vi "ccdIsOpen.vi"() -> ()   [LabVIEW 2023, in "CCD.lvclass"]
uses:
  CCD.lvclass
  CCD.lvclass/CCD.ctl
  d9b87029-586e-44ee-a6e5-d4a5e0edce38.vi
  Communicator/Communicator.lvclass
  b59fd1e7-dcda-425c-bd6c-61aafb79e7f4.vi
  GenericDevice/GenericDevice.lvclass
  ccdIsOpen.ctl
panel:
  out "CCD is open?":T1
  out "CCD out":refnum<class "CCD.lvclass">
  in  "CCD in":refnum<class "CCD.lvclass">
  out "error out":errorcluster
  in  "error in (no error)":errorcluster
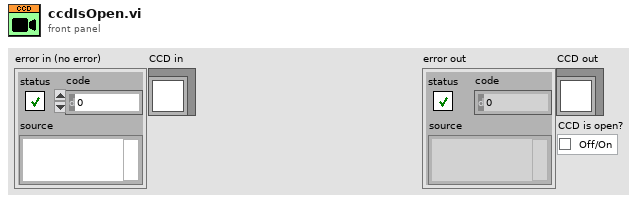
[diagram p1: front panel]
types:
  T1 = typedef "CCD.lvclass/ccdIsOpen.ctl" = cluster{"Checkbox":bool}
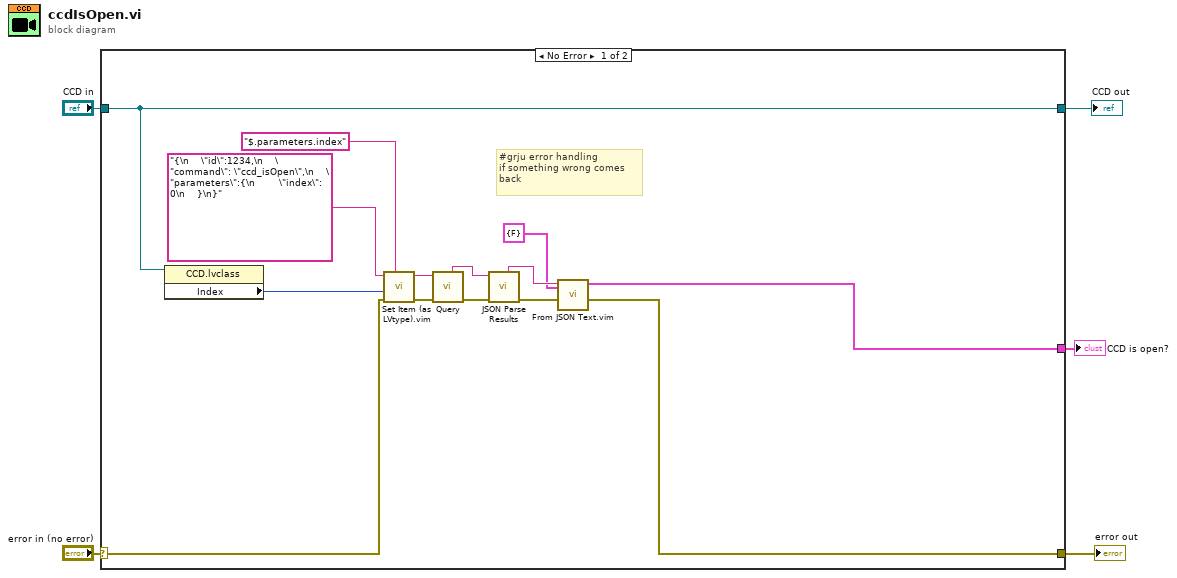
[diagram p0: block diagram]
diagram:
  n1 = case shown="No Error" "error in (no error)" {
    selector: "error in (no error)" -> [w15 w21]
    tunnel: [w12 w21] -> w4
    tunnel: [w17 w20] -> w2
    tunnel: "CCD in" -> [w17 w20]
    tunnel: [w14 _] -> w1
    frame No Error {
      # "#grju error handling\nif something wrong comes\nback"
      n2 = property class="CCD.lvclass"(reference=w17) -> ("Index"=w16:i32)  [unwired: 1 in, 2 out]
      n3 = call "Set Item (as LVtype).vim"("$Path or Item Name"="$.parameters.index", "error in (no error)"=w15, "Anything"=w16, "JSON"="{\n    \"id\":1234,\n    \"command\": \"ccd_isOpen\",\n    \"parameters\":{\n        \"index\": 0\n    }\n}") -> ("error out"=w9:errorcluster, "<JSON>"=w11:string)  [unwired: 4 in, 1 out]
      n4 = call "Query.vi"("error in (no error)"=w9, "String to be sent"=w11) -> ("error out"=w8:errorcluster, "answer from device"=w10:string)  [unwired: 5 in, 3 out]
      n5 = call "JSON Parse Results.vi"("error in (no error)"=w8, "JSON"=w10) -> ("error out"=w13:errorcluster, "results-JSON string"=w7:string)  [unwired: 5 in, 3 out]
      n6 = call "From JSON Text.vim"("Data Type and Default Value"=T1 {"Checkbox"=FALSE} ("Cluster"), "error in (no error)"=w13, "JSON"=w7) -> ("error out"=w12:errorcluster, "Data out"=w14:T1)  [unwired: 7 in]
    }
    frame Error {
    }
  }
  "error out" <- w4
  "CCD out" <- w2
  "CCD is open?" <- w1
